vi "convert--tour to string (in rows).vi"(1 "tour":T1[](array[typedef])) -> (0 "tour (string)":string)   [LabVIEW 2020, in "main.lvlib"]
uses:
  main.lvlib
  core/core_data/chessboard_index.ctl
  core/core.lvlib
  core/core_data/core_data.lvlib
panel:
  out "one square":string
  out "T = not last element in row":bool
  out "square number (prefix)":i32
  out "A row of up to nelements":T1[](array[typedef])
  out "T = not last row":bool
  out "m = no. of rows":i32
  # "Development\ncontrols/indicators useful for development and testing, but which are not outputs of the VI"
  # "Input\nInputs to the VI"
  # "Output\nOutputs of the VI"
  # "Description\n\nBlank VI with error handling case. \n\nSummarize the use of this VI in this space."
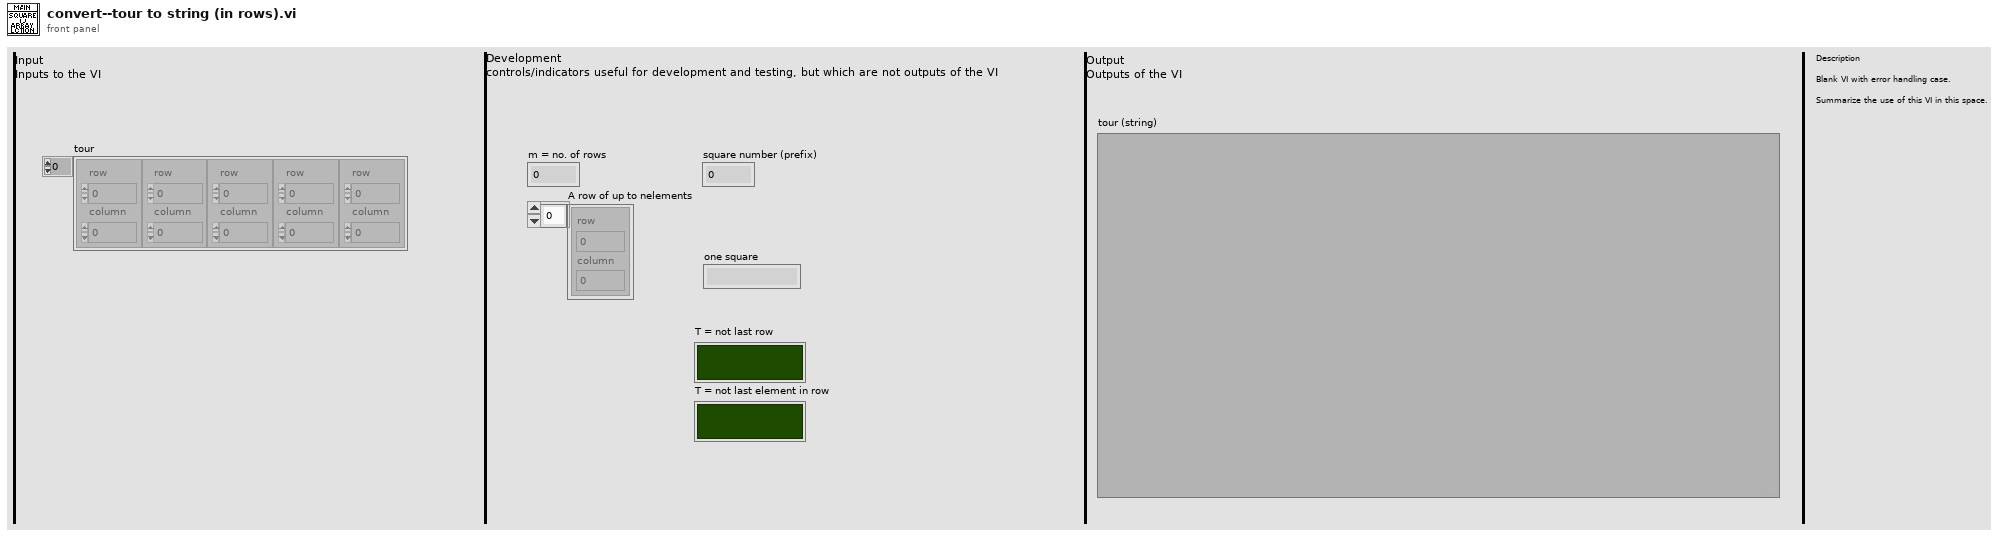
[diagram p1: front panel]
types:
  T1 = typedef "core.lvlib/core_data.lvlib/chessboard_index.ctl" = cluster{"row":u8, "column":u8}
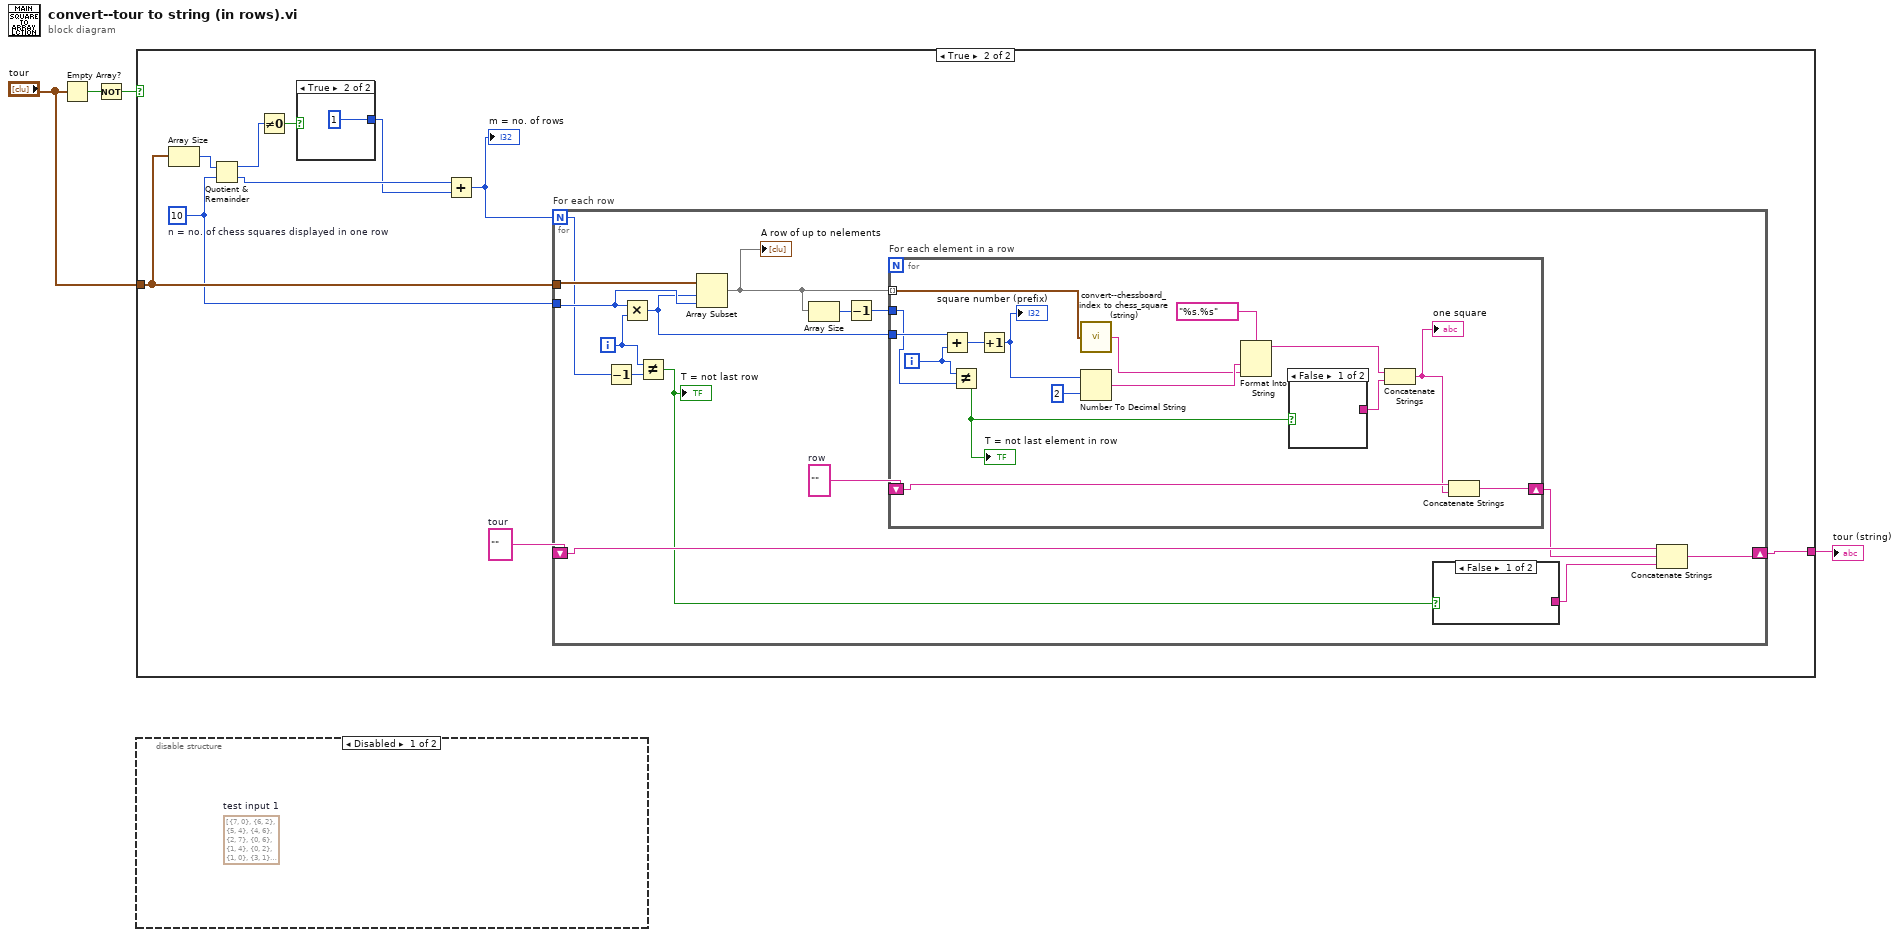
[diagram p0: block diagram]
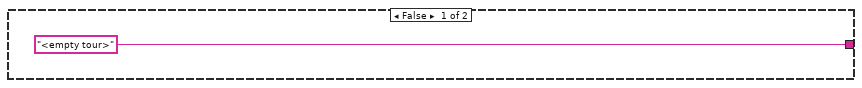
[diagram p3: hidden frame]
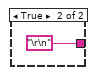
[diagram p5: hidden frame]
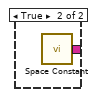
[diagram p6: hidden frame]
diagram:
  n1 = Empty Array?(array="tour") -> (empty?=w4:bool)
  n2 = Not(x=w4) -> (.not. x?=w3:bool)
  n3 = case shown="True" w3 {
    tunnel: ["<empty tour>" w6] -> w2
    tunnel: "tour" -> [_ w14]
    frame False {
    }
    frame True {
      w7 = 10  # n = no. of chess squares displayed in one row
      w15 = ""  # tour
      n4 = Array Size(array=w14) -> (size(s)=w13:i32)
      n5 = Quotient & Remainder(x=w13, y=w7) -> (x-y*floor(x/y)=w12:i32, floor(x/y)=w11:i32)
      n6 = Not Equal To 0?(x=w12) -> (x != 0?=w10:bool)
      n7 = case shown="True" w10 {
        tunnel: [_ 1 ("y")] -> w9
        frame False {
        }
        frame True {
        }
      }
      n8 = Add(x=w11, y=w9) -> (x+y=w8:i32)
      "m = no. of rows" <- w8
      n9 = for "For each row" {
        N: w8 -> [w27]
        tunnel: w14 -> [w31]
        tunnel: w7 -> [w30]
        shift-right: [w17] -> w6
        shift-left: w15 -> [w21]
        i -> [w29]
        w26 = ""  # row
        n10 = Decrement(x=w27) -> (x-1=w28:i32)
        n11 = Multiply(x=w30, y=w29) -> (x*y=w25:i32)
        n12 = Not Equal?(x=w29, y=w28) -> (x != y?=w19:bool)
        "T = not last row" <- w19
        n13 = Array Subset(array=w31, index=w25, length=w30) -> (w24:T1[])
        "A row of up to nelements" <- w24
        n14 = Array Size(array=w24) -> (size(s)=w23:i32)
        n15 = Decrement(x=w23) -> (x-1=w22:i32)
        n16 = for "For each element in a row" {
          tunnel: w25 -> [w48]
          tunnel: w24 -> [w46] mode=indexing
          tunnel: w22 -> [w39]
          shift-right: [w33] -> w20
          shift-left: w26 -> [w35]
          i -> [w40]
          n17 = Add(x=w48, y=w40) -> (x+y=w47:i32)
          n18 = Not Equal?(x=w40, y=w39) -> (x != y?=w36:bool)
          "T = not last element in row" <- w36
          n19 = Increment(x=w47) -> (x+1=w44:i32)
          "square number (prefix)" <- w44
          n20 = call "convert--chessboard_index to chess_square (string).vi"("chessboard_index"=w46) -> ("chess square (string)"=w37:string)
          n21 = Number To Decimal String(number=w44, width (-)=i16 2) -> (decimal integer string=w38:string)
          n22 = Format Into String(format string="%s.%s", w38, w37) -> (resulting string=w42:string)  [unwired: 2 in, 1 out]
          n23 = case shown="False" w36 {
            tunnel: [_ w49] -> w41
            frame False {
            }
            frame True {
              n24 = call <vilib>:"Space Constant.vi"() -> ("String"=w49:string)
            }
          }
          n25 = Concatenate Strings(w42, w41) -> (w34:string)
          "one square" <- w34
          n26 = Concatenate Strings(w35, w34) -> (w33:string)
        }
        n27 = case shown="False" w19 {
          tunnel: [_ "\r\n"] -> w18
          frame False {
          }
          frame True {
          }
        }
        n28 = Concatenate Strings(w21, w20, w18) -> (w17:string)
      }
    }
  }
  "tour (string)" <- w2
  n29 = disable-structure shown="Disabled" {
    frame Disabled {
      (unwired) T1[] [{"row"=7, "column"=0}, {"row"=6, "column"=2}, {"row"=5, "column"=4}, {"row"=4, "column"=6}, {"row"=2, "column"=7}, {"row"=0, "column"=6}, {"row"=1, "column"=4}, {"row"=0, "column"=2}, {"row"=1, "column"=0}, {"row"=3, "column"=1}, {"row"=2, "column"=3}, {"row"=1, "column"=5}, {"row"=0, "column"=7}, {"row"=2, "column"=6}, {"row"=0, "column"=5}, {"row"=1, "column"=3}, {"row"=0, "column"=1}, {"row"=2, "column"=0}, {"row"=1, "column"=2}, {"row"=0, "column"=4}, {"row"=2, "column"=5}, {"row"=1, "column"=7}, {"row"=3, "column"=6}, {"row"=2, "column"=4}, {"row"=1, "column"=6}, {"row"=3, "column"=5}, {"row"=4, "column"=3}, {"row"=2, "column"=2}, {"row"=0, "column"=3}, {"row"=1, "column"=1}, {"row"=3, "column"=0}, {"row"=5, "column"=1}, {"row"=3, "column"=2}]  # test input 1
    }
    frame Enabled {
    }
  }
